vi "AutoDistance.vi"(6 "error in (no error)":errorcluster, 7 "Mode":T1, 8 "Slowdown":dbl format="%#_13g", 9 "Brake":dbl format="%#_13g", 10 "DesiredDistance":dbl format="%#_13g", 11 "CurrentDistance":dbl format="%#_13g") -> (1 "TankDriveRight":dbl, 2 "TankDriveLeft":dbl, 3 "Finished":bool=TRUE, 4 "error out":errorcluster)   [LabVIEW 2013]
doc: "Determines the motor inputs needed for the left and right sides of tank drive to reach the distance setpoint.\n-Mode: fullspeed (i.e. floor it until the robot gets there) or linear (linear relation between distance to go and motor input).\n-DesiredDistance: the setpoint distance\n-CurrentDistance: the current distance to the target\n-Brake: the minimum distance from the setpoint the robot needs to be in order to brake\n-Slowdown: the maximum distance from the setpoint at which the robot can go full speed"
uses:
  AutoAlignMode.ctl
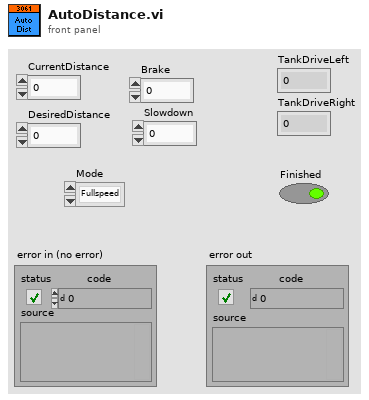
[diagram p1: front panel]
types:
  T1 = typedef "AutoAlignMode.ctl" = enum16{"Fullspeed", "Linear"}
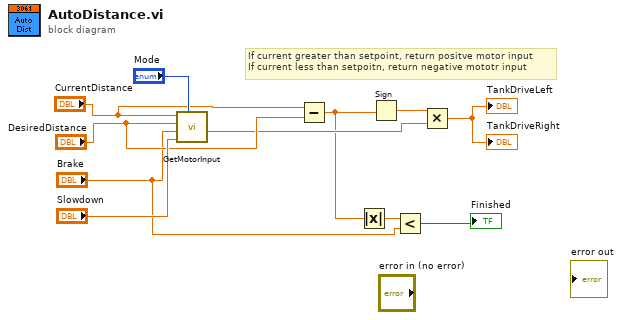
[diagram p0: block diagram]
diagram:
  # "If current greater than setpoint, return positve motor input\nIf current less than setpoitn, return negative mototr input"
  n1 = call "GetMotorInput.vi"("Mode"="Mode", "Slowdown"="Slowdown", "Brake"="Brake", "Setpoint"="DesiredDistance", "Current"="CurrentDistance") -> ("MotorInput"=w6:dbl)  [unwired: 6 in]
  n2 = Subtract(x="CurrentDistance", y="DesiredDistance") -> (x-y=w4:dbl)
  n3 = Absolute Value(x=w4) -> (abs(x)=w3:dbl)
  n4 = Sign(1:w4) -> (0:w7:dbl)
  n5 = Less?(x=w3, y="Brake") -> (x < y?=→"Finished":bool)
  n6 = Multiply(x=w7, y=w6) -> (x*y=→"TankDriveLeft" →"TankDriveRight":dbl)
